vi "Eliminated.vi"(6 "Column":i32, 8 "Row":i32, 9 "Killer":i32, 10 "Team":i32, 11 "Hail in":refnum<class "Hail.lvclass">) -> (3 "Hail out":refnum<class "Hail.lvclass">)   [LabVIEW 2015, in "Hail.lvclass"]
uses:
  Hail.lvclass
  Hail.lvclass/Hail.ctl
  Square/Square.lvclass
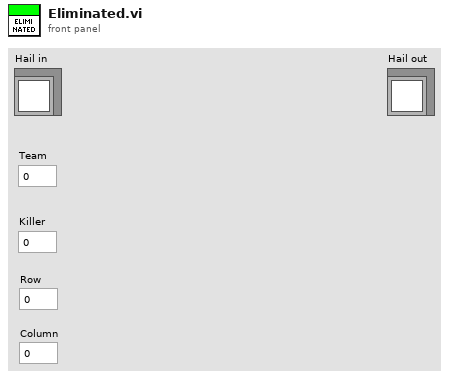
[diagram p1: front panel]
types:
  T1 = typedef "Hail.lvclass/Board Cluster.ctl" = cluster{"Group[][]":i32[][], "Center":cluster{"Col":i32, "Row":i32}, "Spread Dist":i32, "Radius Idx":i32, "Circum Idx":i32, "Attractor[][]":i32[][]}
  T2 = typedef "Hail.lvclass/Group Cluster.ctl" = cluster{"Mode":T3, "Move Amt":i32, "Group Cnt":i32, "Temp":u32, "Round":i32}
  T3 = typedef "Hail.lvclass/Mode Enum.ctl" = enum16{"Grow(1)", "Grow(2)", "Grow(4)", "Grow(8)", "Divide", "Farewell", "Move"}
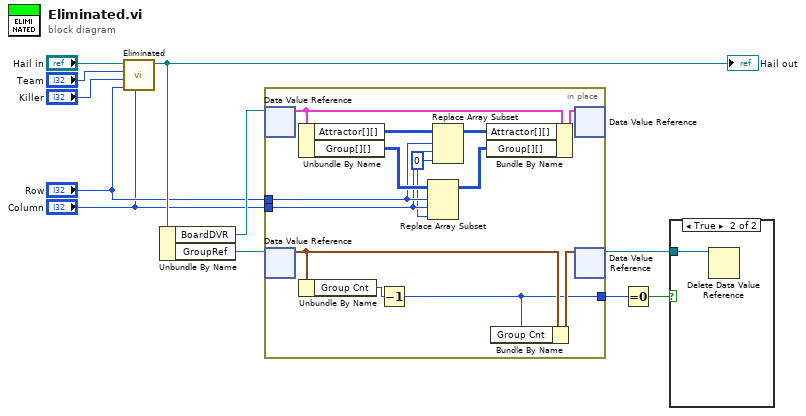
[diagram p0: block diagram]
diagram:
  n1 = call-parent "Eliminated.vi"("Column"="Column", "Row"="Row", "Killer"="Killer", "Team"="Team", "Square in"="Hail in") -> ("Square out"=w7:refnum<class "Hail.lvclass">)  [unwired: 6 in]
  "Hail out" <- w7
  n2 = Unbundle By Name(w7) -> ("BoardDVR"=w3:refnum<data-value>, "GroupRef"=w8:refnum<data-value>)
  n3 = in-place {
    in-place-border: [w21] -> w6
    in-place-border: "Row" -> [w14]
    in-place-border: "Column" -> [w13]
    w12 = 0 ("new element/subarray")
    n4 = in-place-dvr #1(w3) -> (w20:T1)  [unwired: 1 out]
    n5 = in-place-dvr #2(w8) -> (w24:T2)  [unwired: 1 out]
    n6 = Unbundle By Name(w20) -> ("Attractor[][]"=w18:i32[][], "Group[][]"=w16:i32[][])
    n7 = Unbundle By Name(w24) -> ("Group Cnt"=w23:i32)
    n8 = Decrement(x=w23) -> (x-1=w21:i32)
    n9 = Replace Array Subset(array=w16, new element=w12, index (row)=w14, index (col)=w13) -> (w15:i32[][])
    n10 = Replace Array Subset(array=w18, new element=w12, index (row)=w14, index (col)=w13) -> (w17:i32[][])
    n11 = Bundle By Name(cluster=w20, "Attractor[][]"=w17, "Group[][]"=w15) -> (w19:T1)
    n12 = Bundle By Name(cluster=w24, "Group Cnt"=w21) -> (w22:T2)
    n13 = in-place-dvr #1(w19) -> ()  [unwired: 2 out]
    n14 = in-place-dvr #2(w22) -> (w5:refnum<data-value>)  [unwired: 1 out]
  }
  n15 = Equal To 0?(x=w6) -> (x = 0?=w4:bool)
  n16 = case shown="True" w4 {
    tunnel: w5 -> [_ w25]
    frame False {
    }
    frame True {
      n17 = Delete Data Value Reference(data value reference=w25) -> ()  [unwired: 1 in, 2 out]
    }
  }
